vi "Write Send Text Data.vi"(8 "error in (no error)":errorcluster, 9 "values":string, 10 "starting address":u16, 11 "standard data model in":refnum<class "WebSocket Data Model.lvclass">) -> (0 "error out":errorcluster, 3 "standard data model out":refnum<class "WebSocket Data Model.lvclass">)   [LabVIEW 2021, in "WebSockets.lvlib" / "WebSocket Data Model.lvclass"]
doc: "Writes the values of multiple input register values in series, starting at address M."
uses:
  WebSocket Data Model.lvclass
  WebSocket Data Model.lvclass/WebSocket Data Model.ctl
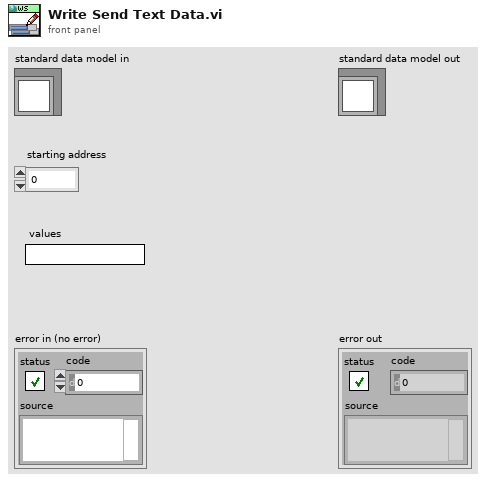
[diagram p1: front panel]
types:
  T1 = typedef "WebSockets.lvlib/WebSocket Data Model.lvclass/Data Model.ctl" = cluster{"UTC":u64, "Receive Binary Data":u8[], "Receive Text Data":string, "Send Binary Data":u8[], "Send Text Data":string, "ES":u8}
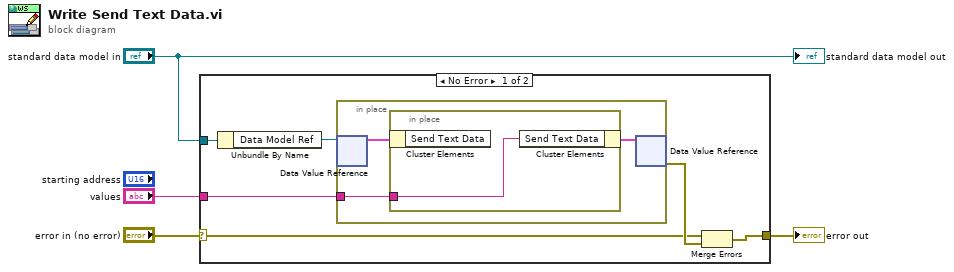
[diagram p0: block diagram]
diagram:
  n1 = case shown="No Error" "error in (no error)" {
    selector: "error in (no error)" -> [w5 w15]
    tunnel: "values" -> [w10 _]
    tunnel: "standard data model in" -> [w9 _]
    tunnel: [w8 w15] -> w2
    frame No Error {
      n2 = Unbundle By Name(w9) -> ("Data Model Ref"=w7:refnum<data-value>)
      n3 = in-place {
        in-place-border: w10 -> [w13]
        n4 = in-place-dvr #1(w7) -> (w12:T1)  [unwired: 1 out]
        n5 = in-place {
          in-place-border: w13 -> [w14]
          n6 = in-place-cluster #2(w12) -> ()  [unwired: 1 out]
          n7 = in-place-cluster #2("Send Text Data"=w14) -> (w11:T1)
        }
        n8 = in-place-dvr #1(w11) -> (w6:errorcluster)  [unwired: 1 out]
      }
      n9 = Merge Errors(w5, w6) -> (w8:errorcluster)
    }
    frame Error {
    }
  }
  "error out" <- w2
  "standard data model out" <- "standard data model in"
